vi "prepare_and_save.vi"(8 "error in (no error)":errorcluster, 10 "array with duplicates removed":string[](array[string]), 11 "Array":i32[](array[numeric])) -> (0 "error out":errorcluster)   [LabVIEW 2020]
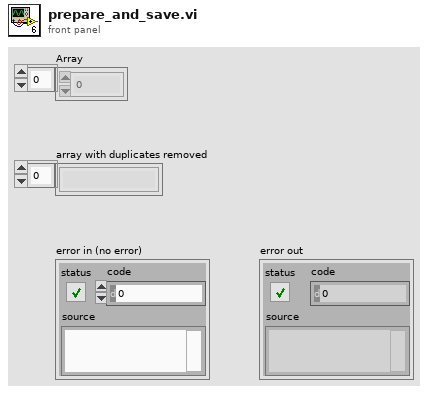
[diagram p1: front panel]
types:
  T1 = enum16{"open", "replace", "create", "open or create", "replace or create", "replace or create with confirmation"}
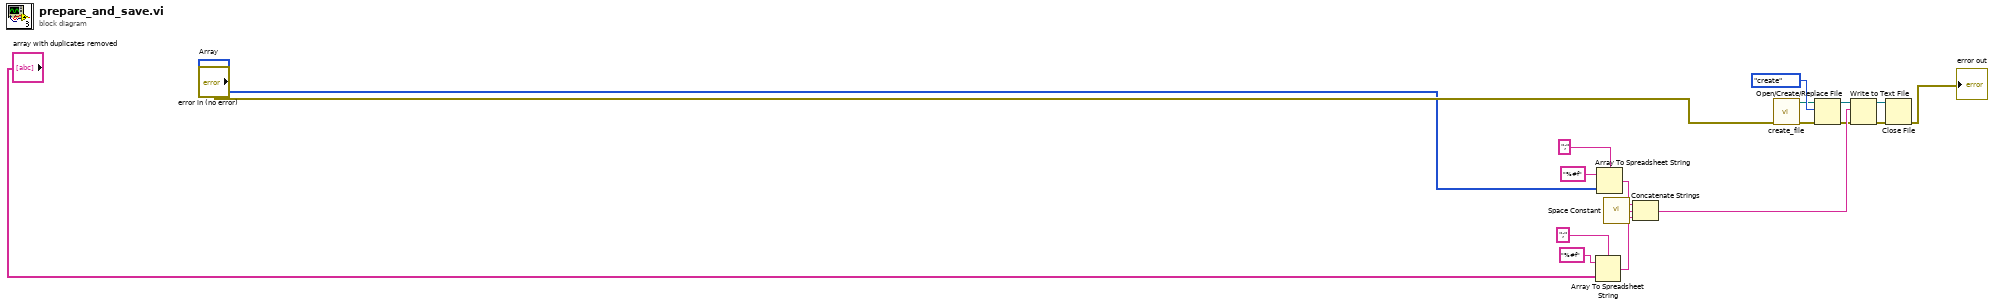
[diagram p0: block diagram]
diagram:
  n1 = Array To Spreadsheet String(delimiter (Tab)=";", array="array with duplicates removed", 3:"%#f" ("format string")) -> (spreadsheet string=w14:string)
  n2 = Array To Spreadsheet String(delimiter (Tab)=";", array="Array", 3:"%#f" ("format string")) -> (spreadsheet string=w13:string)
  n3 = call <vilib>:"Space Constant.vi"() -> ("String"=w16:string)
  n4 = Concatenate Strings(w13, w16, w14) -> (w15:string)
  n5 = call "create_file.vi"("error in (no error)"="error in (no error)") -> ("error out"=w6:errorcluster, "appended path"=w5:path)  [unwired: 9 in]
  n6 = Open/Create/Replace File(file path (use dialog)=w5, error in=w6, operation (0:open)=T1."create") -> (refnum out=w1:refnum<file>, error out=w2:errorcluster)  [unwired: 3 in, 1 out]
  n7 = Write to Text File(file (use dialog)=w1, text=w15, error in=w2) -> (refnum out=w3:refnum<file>, error out=w4:errorcluster)  [unwired: 1 in, 1 out]
  n8 = Close File(refnum=w3, error in=w4) -> (error out=→"error out":errorcluster)  [unwired: 1 out]
